vi "Clear Config for Active.vi"(8 "error in (no error)":errorcluster, 11 "Cfg Grandmaster in":refnum<class "Cfg Grandmaster.lvclass">) -> (0 "error out":errorcluster, 3 "Cfg Grandmaster out":refnum<class "Cfg Grandmaster.lvclass">)   [LabVIEW 2012, in "Configuration Grandmaster.lvlib" / "Cfg Grandmaster.lvclass"]
uses:
  Cfg Grandmaster.lvclass
  Cfg Grandmaster.lvclass/Cfg Grandmaster.ctl
  Class Chassis BOM/Chassis BOM.lvclass/Chassis BOM.ctl
  Class Chassis BOM/Read ChassisType.vi
  Class Chassis BOM/Read Chassis Alias.vi
  Class Chassis BOM/Write CfgFile.vi
  Class Chassis Cfg/ChassisCfg.lvclass
  Class Chassis BOM/Chassis BOM.lvclass
  Class FP Ctrls/FP Controls.lvclass
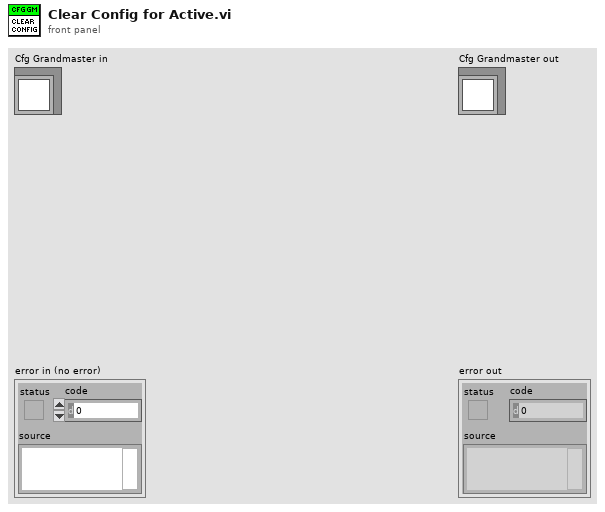
[diagram p1: front panel]
types:
  T1 = typedef "ge_Cfg wChassis.ctl" = cluster{"Chassis BOM":refnum<class "Chassis BOM.lvclass">, "Chassis Cfg":refnum<class "ChassisCfg.lvclass">, "Chassis Tasks":refnum<class "Chassis Tasks.lvclass">, "HW Error":bool, "Unsvd Chgs?":bool}
  T2 = typedef "Chassis Type.ctl" = enum16{"Not Supported", "C Series 1-Slot", "C Series 4-Slot", "C Series 8-Slot", "PXI 8-Slot", "PXIe 18-Slot"}
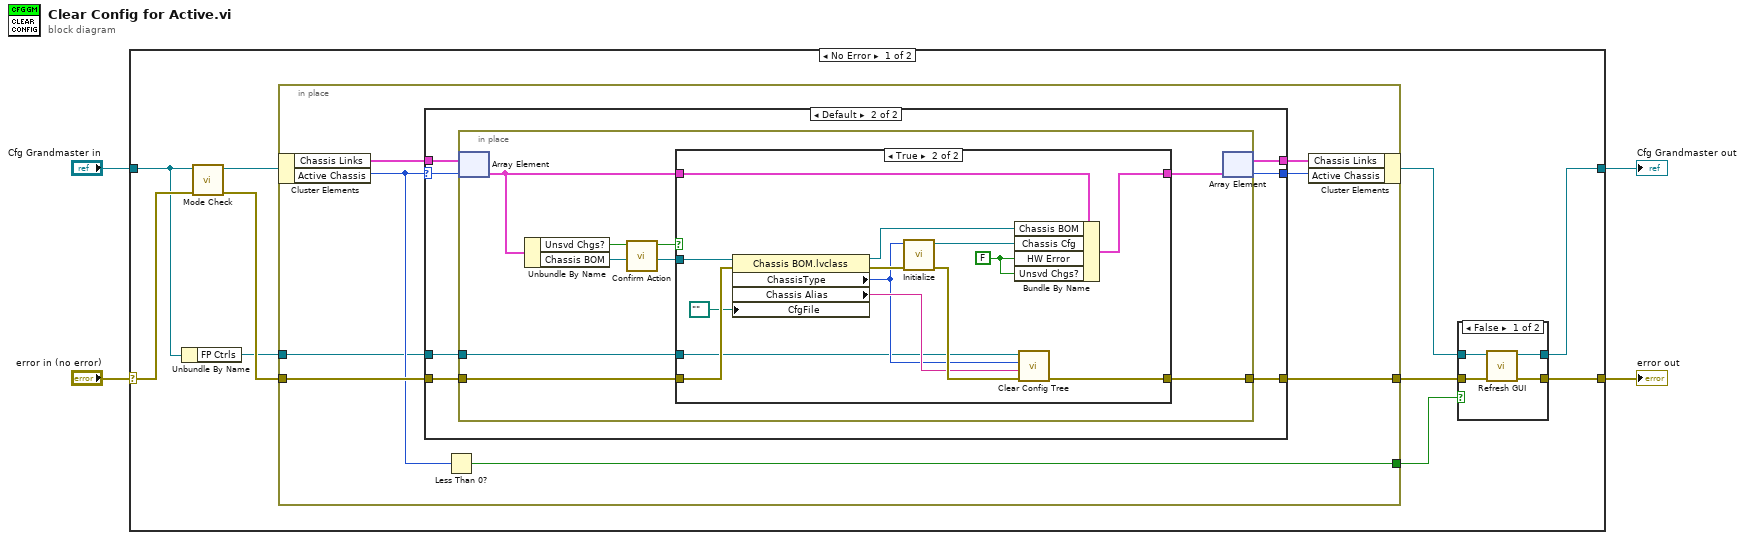
[diagram p0: block diagram]
diagram:
  n1 = case shown="No Error" "error in (no error)" {
    selector: "error in (no error)" -> [w12 w64]
    tunnel: [w10 w64] -> w3
    tunnel: [w8 w63] -> w1
    tunnel: "Cfg Grandmaster in" -> [w6 w63]
    frame No Error {
      n2 = Unbundle By Name(w6) -> ("FP Ctrls"=w5:refnum<class "FP Controls.lvclass">)
      n3 = call "Mode Check.vi"("error in (no error)"=w12, "Cfg Grandmaster in"=w6) -> ("error out"=w13:errorcluster, "Cfg Grandmaster out"=w14:refnum<class "Cfg Grandmaster.lvclass">)  [unwired: 8 in]
      n4 = in-place {
        in-place-border: [w28] -> w11
        in-place-border: w13 -> [w27]
        in-place-border: [w24] -> w7
        in-place-border: w5 -> [w21]
        n5 = in-place-cluster #1(w14) -> ("Chassis Links"=w26:T1[], "Active Chassis"=w23:i32)
        n6 = case shown="Default" w23 {
          selector: w23 -> [w29 w34]
          tunnel: [w31 w38] -> w25
          tunnel: w26 -> [w31 w37]
          tunnel: w27 -> [w30 w36]
          tunnel: [w30 w35] -> w28
          tunnel: [w29 w33] -> w22
          tunnel: w21 -> [_ w32]
          frame -1 {
          }
          frame Default {
            n7 = in-place {
              in-place-border: w36 -> [w42]
              in-place-border: [w44] -> w35
              in-place-border: w32 -> [w39]
              n8 = in-place-array #2(w37, w34) -> (w45:T1)
              n9 = Unbundle By Name(w45) -> ("Unsvd Chgs?"=w41:bool, "Chassis BOM"=w43:refnum<class "Chassis BOM.lvclass">)
              n10 = call "Confirm Action.vi"("Confirm?"=w41) -> ("T button?"=w40:bool)  [unwired: 10 in]
              n11 = case shown="True" w40 {
                tunnel: [w48 w61] -> w46
                tunnel: w45 -> [w48 w59]
                tunnel: [w47 w52] -> w44
                tunnel: w43 -> [_ w58]
                tunnel: w42 -> [w47 w56]
                tunnel: w39 -> [_ w49]
                frame False {
                }
                frame True {
                  w62 = FALSE ("HW Error")
                  n12 = property class="Chassis BOM.lvclass"(reference=w58, error in=w56, "CfgFile"=path "") -> (reference out=w55:refnum<class "Chassis BOM.lvclass">, error out=w57:errorcluster, "ChassisType"=w50:T2, "Chassis Alias"=w51:string)
                  n13 = call "Initialize.vi"("error in"=w57, "ChassisType"=w50) -> ("error out"=w53:errorcluster, "Chassis Cfg"=w60:refnum<class "ChassisCfg.lvclass">)  [unwired: 7 in]
                  n14 = Bundle By Name(cluster=w59, "Chassis BOM"=w55, "Chassis Cfg"=w60, "HW Error"=w62, "Unsvd Chgs?"=w62) -> (w61:T1)
                  n15 = call "Clear Config Tree.vi"("error in"=w53, "Chassis Name"=w51, "ChassisType"=w50, "FP Controls in"=w49) -> ("error out"=w52:errorcluster)  [unwired: 6 in, 1 out]
                }
              }
              n16 = in-place-array #2(w46) -> (w38:T1[], w33:i32)
            }
          }
        }
        n17 = Less Than 0?(x=w23) -> (x < 0?=w24:bool)
        n18 = in-place-cluster #1("Chassis Links"=w25, "Active Chassis"=w22) -> (w9:refnum<class "Cfg Grandmaster.lvclass">)
      }
      n19 = case shown="False" w7 {
        tunnel: [w17 w20] -> w10
        tunnel: w11 -> [w18 w20]
        tunnel: w9 -> [w16 w19]
        tunnel: [w15 w19] -> w8
        frame False {
          n20 = call "Refresh GUI.vi"("error in (no error)"=w18, "Cfg Grandmaster in"=w16) -> ("error out"=w17:errorcluster, "Cfg Grandmaster out"=w15:refnum<class "Cfg Grandmaster.lvclass">)  [unwired: 8 in]
        }
        frame True {
        }
      }
    }
    frame Error {
    }
  }
  "error out" <- w3
  "Cfg Grandmaster out" <- w1
